vi "Read Matlab Params.vi"(8 "error in (no error)":errorcluster, 10 "Enum":T1(ring), 11 "TrialBasedExperiment in":refnum<class "DotMapping.lvclass">) -> (0 "error out":errorcluster, 2 "Matlab Param Array":cluster{"Name":string, "Data":variant}[](array[cluster]), 3 "TrialBasedExperiment out":refnum<class "DotMapping.lvclass">)   [LabVIEW 2010]
uses:
  DotMapping.lvclass
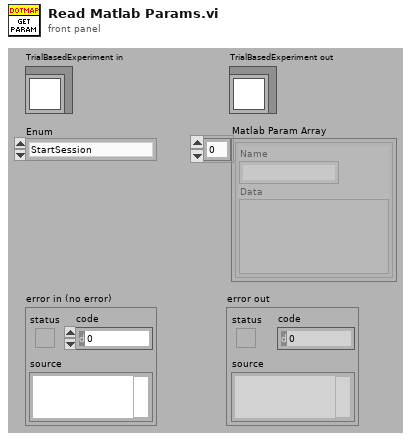
[diagram p1: front panel]
types:
  T1 = enum16{"StartSession", "StartTrial", "ShowStimulus"}
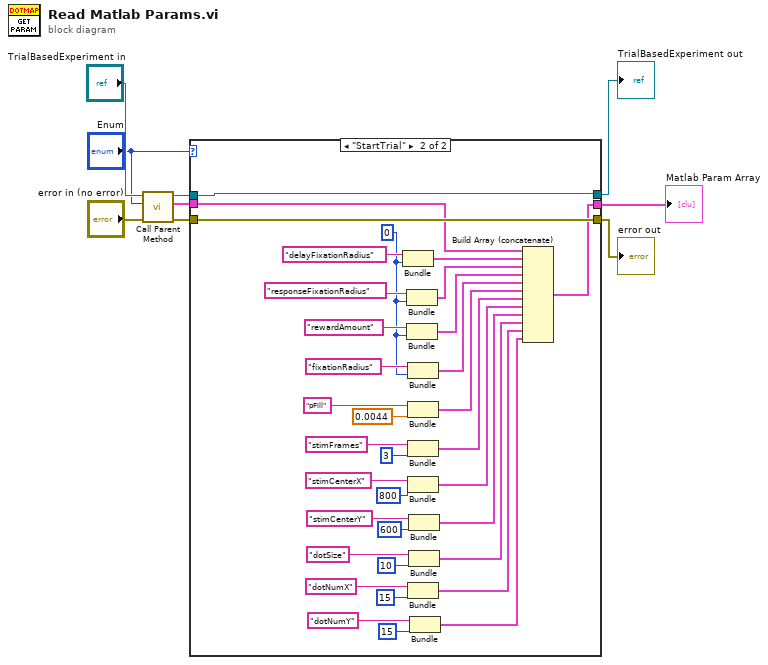
[diagram p0: block diagram]
diagram:
  n1 = call-parent "Call Parent Method"("error in (no error)"="error in (no error)", "Enum"="Enum", "TrialBasedExperiment in"="TrialBasedExperiment in") -> ("error out"=w5:errorcluster, "Matlab Param Array"=w6:cluster{"Name":string, "Data":variant}[], "TrialBasedExperiment out"=w7:refnum<class "DotMapping.lvclass">)  [unwired: 6 in]
  n2 = case shown="\"StartTrial\"" "Enum" {
    tunnel: w7 -> [w12 w39]
    tunnel: w5 -> [w11 w46]
    tunnel: [w12 w39] -> w3
    tunnel: w6 -> [w10 w44]
    tunnel: [w11 w46] -> w1
    tunnel: [w10 w42] -> w2
    frame "StartSession", Default {
    }
    frame "StartTrial" {
      w34 = 0
      n3 = Bundle("delayFixationRadius", w34) -> (w43:cluster{string, i32})  [unwired: 1 out]
      n4 = Bundle("responseFixationRadius", w34) -> (w40:cluster{string, i32})  [unwired: 1 out]
      n5 = Bundle("rewardAmount", w34) -> (w37:cluster{string, i32})  [unwired: 1 out]
      n6 = Bundle("fixationRadius", w34) -> (w35:cluster{string, i32})  [unwired: 1 out]
      n7 = Bundle("pFill", 0.0044) -> (w19:cluster{string, dbl})  [unwired: 1 out]
      n8 = Bundle("stimFrames", 3) -> (w18:cluster{string, i32})  [unwired: 1 out]
      n9 = Bundle("stimCenterX", 800) -> (w17:cluster{string, i32})  [unwired: 1 out]
      n10 = Bundle("dotNumX", 15) -> (w14:cluster{string, i32})  [unwired: 1 out]
      n11 = Bundle("stimCenterY", 600) -> (w16:cluster{string, i32})  [unwired: 1 out]
      n12 = Bundle("dotSize", 10) -> (w15:cluster{string, i32})  [unwired: 1 out]
      n13 = Bundle("dotNumY", 15) -> (w13:cluster{string, i32})  [unwired: 1 out]
      n14 = Build Array (concatenate)(w44, w43, w40, w37, w35, w19, w18, w17, w16, w15, w14, w13) -> (w42:cluster{"Name":string, "Data":variant}[])
    }
  }
  "error out" <- w1
  "TrialBasedExperiment out" <- w3
  "Matlab Param Array" <- w2
